vi "MALT Set One.vi"(8 "error in":errorcluster, 9 "Port":i32, 10 "Address":i32, 11 "CardType":i32) -> (0 "error out":errorcluster)   [LabVIEW 2018]
panel:
  out "data out":string
  out "request command":string
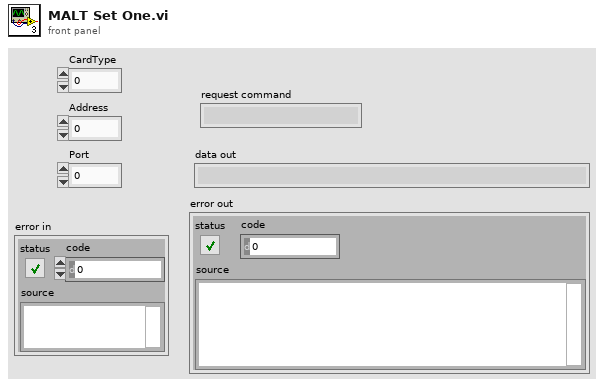
[diagram p1: front panel]
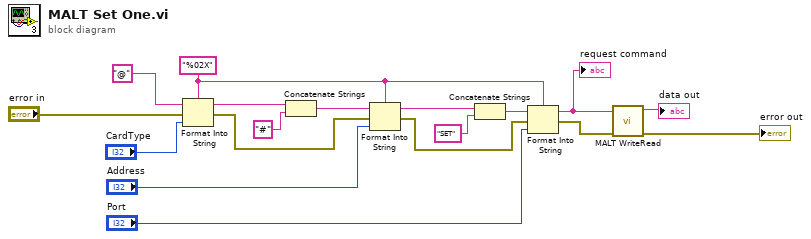
[diagram p0: block diagram]
diagram:
  w6 = "%02X" ("format string")
  n1 = Format Into String(format string=w6, initial string="@", error in="error in", "CardType") -> (resulting string=w16:string, error out=w10:errorcluster)
  n2 = Concatenate Strings(w16, "#" ("string")) -> (w14:string)
  n3 = Format Into String(format string=w6, initial string=w14, error in=w10, "Address") -> (resulting string=w11:string, error out=w8:errorcluster)
  n4 = Concatenate Strings(w11, "SET" ("resulting string")) -> (w9:string)
  n5 = Format Into String(format string=w6, initial string=w9, error in=w8, "Port") -> (resulting string=w5:string, error out=w4:errorcluster)
  "request command" <- w5
  n6 = call "MALT WriteRead.vi"("error in"=w4, "data in"=w5) -> ("error out"=→"error out":errorcluster, "data out"=→"data out":string)  [unwired: 8 in]
